vi "Write Date to SnP File.vi"(0 "Result File Path In":path, 5 "Date":timestamp, 11 "error in":errorcluster) -> (4 "Result File Path Out":path, 15 "error out":errorcluster)   [LabVIEW 2023, in "RFFixtureCharact.RFPM.lvlib" / "Charact Result Accessor.lvclass"]
uses:
  Charact Result Accessor.lvclass
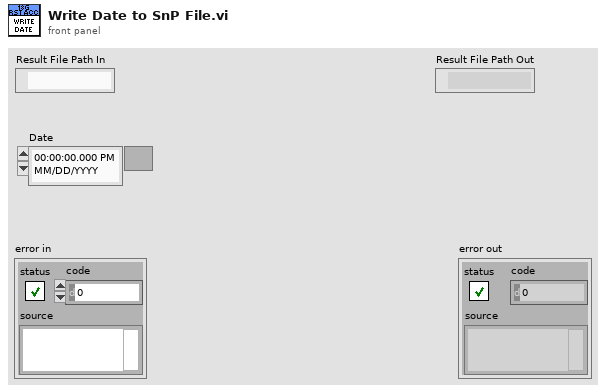
[diagram p1: front panel]
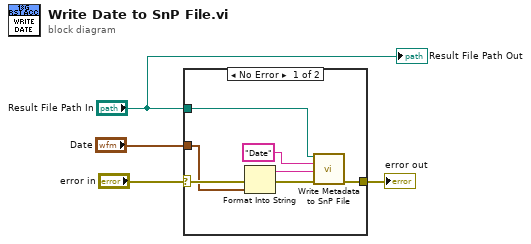
[diagram p0: block diagram]
diagram:
  n1 = case shown="No Error" "error in" {
    selector: "error in" -> [w6 w12]
    tunnel: [w10 w12] -> w3
    tunnel: "Result File Path In" -> [w7 _]
    tunnel: "Date" -> [w5 _]
    frame No Error {
      n2 = Format Into String(error in=w6, w5) -> (resulting string=w8:string, error out=w11:errorcluster)  [unwired: 2 in]
      n3 = call "Write Metadata to SnP File.vi"("SnP File Path in"=w7, "Key"="Date", "Value"=w8, "error in (no error)"=w11) -> ("error out"=w10:errorcluster)  [unwired: 10 in, 1 out]
    }
    frame Error {
    }
  }
  "error out" <- w3
  "Result File Path Out" <- "Result File Path In"
